vi "REQ Wakeup_help_loop.vi"(8 "error in":errorcluster, 9 "Timeout":i32=-1, 11 "Abstract.lvclass":variant) -> (0 "error out":errorcluster)   [LabVIEW 2021, in "DC PWS.lvlib"]
doc: "_____\nCreated using DQMH Event Scripter 6.1.0.128."
uses:
  DC PWS.lvlib
  REQ Wakeup_help_loop Argument--cluster.ctl
  Class/Abstract/Abstract.lvclass
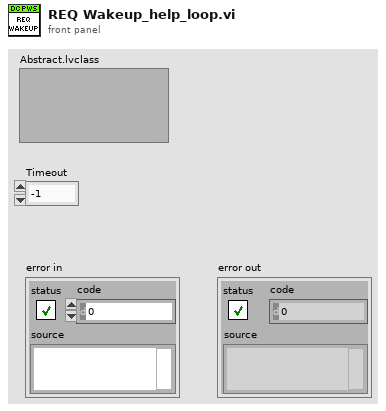
[diagram p1: front panel]
types:
  T1 = typedef "DC PWS.lvlib/REQ Wakeup_help_loop Argument--cluster.ctl" = cluster{"Abstract.lvclass":variant, "Timeout":i32}
  T2 = typedef "DC PWS.lvlib/Request Events--cluster.ctl" = cluster{"Stop Module":refnum<user-event>, "Show Panel":refnum<user-event>, "Hide Panel":refnum<user-event>, "Get Module Execution Status":refnum<user-event>, "Show Diagram":refnum<user-event>, "REQ Initialize Hardware":refnum<user-event>, "REQ Config Current Limit":refnum<user-event>, "REQ Over Voltage Limit":refnum<user-event>, "REQ Configure Output":refnum<user-event>, "REQ Enable Output":refnum<user-event>, "REQ Measurement":refnum<user-event>, "REQ Close Ref":refnum<user-event>, "REQ Wakeup_help_loop":refnum<user-event>, "REQ DC Parameter":refnum<user-event>, "REQ Retry DC PWS":refnum<user-event>}
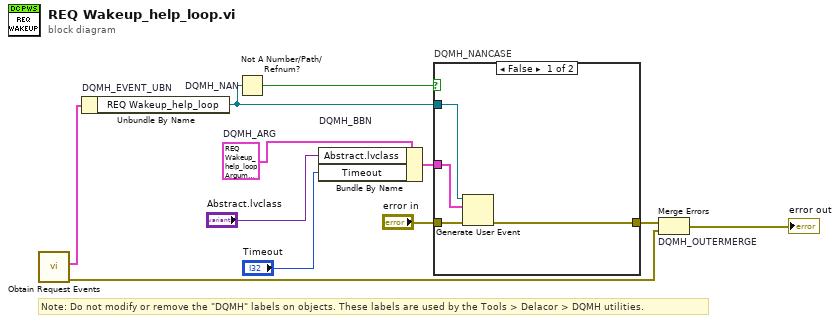
[diagram p0: block diagram]
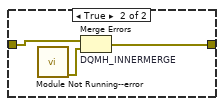
[diagram p2: hidden frame]
diagram:
  w5 = T1 {"Abstract.lvclass"=variant(refnum<class "Abstract.lvclass"> refnum), "Timeout"=-1}  # DQMH_ARG
  # "Note: Do not modify or remove the \"DQMH\" labels on objects. These labels are used by the Tools > Delacor > DQMH utilities."
  n1 = call "Obtain Request Events.vi"() -> ("error out"=w2:errorcluster, "DC PWS Request Events"=w1:T2)  [unwired: 10 in]
  n2 = Unbundle By Name "DQMH_EVENT_UBN"(w1) -> ("REQ Wakeup_help_loop"=w7:refnum<user-event>)
  n3 = Not A Number/Path/Refnum? "DQMH_NAN"(number/path/refnum=w7) -> (NaN/Path/Refnum?=w8:bool)
  n4 = Bundle By Name "DQMH_BBN"(cluster=w5, "Abstract.lvclass"="Abstract.lvclass", "Timeout"="Timeout") -> (w9:T1)
  n5 = case "DQMH_NANCASE" shown="False" w8 {
    tunnel: "error in" -> [w15 w18]
    tunnel: [w14 w17] -> w6
    tunnel: w7 -> [w13 _]
    tunnel: w9 -> [w12 _]
    frame False {
      n6 = Generate User Event(user event=w13, event data cluster=w12, error in=w15) -> (error out=w14:errorcluster)  [unwired: 1 in, 1 out]
    }
    frame True {
      n7 = call "Module Not Running--error.vi"() -> ("error out"=w16:errorcluster)  [unwired: 11 in]
      n8 = Merge Errors "DQMH_INNERMERGE"(w18, w16) -> (w17:errorcluster)
    }
  }
  n9 = Merge Errors "DQMH_OUTERMERGE"(w6, w2) -> (→"error out":errorcluster)
